vi "Initialise.vi"() -> (0 "error out":errorcluster, 3 "axopatch-200B out":refnum<class "axopatch-200B.lvclass">)   [LabVIEW 2014, in "axopatch-200B.lvclass"]
uses:
  axopatch-200B.lvclass
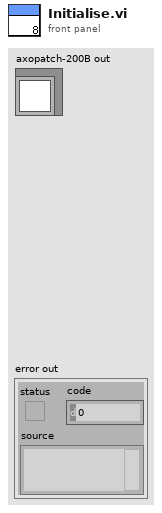
[diagram p1: front panel]
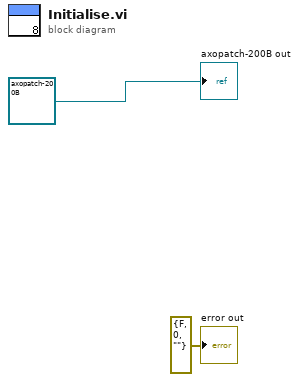
[diagram p0: block diagram]
diagram:
  "error out" <- errorcluster {"status"=FALSE, "code"=0, "source"=""} ("error out")
  "axopatch-200B out" <- refnum<class "axopatch-200B.lvclass"> refnum ("axopatch-200B out")
